vi "Update Fields Table for Spartan 3.0.vi"(8 "error in":errorcluster, 11 "Connection Refnum In":T1) -> (0 "error out":errorcluster, 3 "Connection Refnum Out":T1)   [LabVIEW 2011]
uses:
  Field Record.ctl
  Field DataTypes.ctl
  Field NextItem.ctl
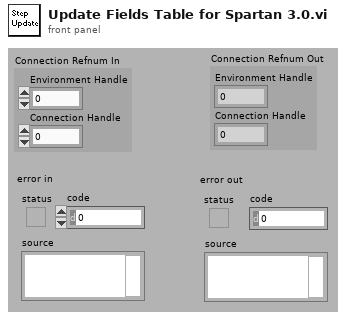
[diagram p1: front panel]
types:
  T1 = cluster{"Environment Handle":i32, "Connection Handle":i32}
  T2 = typedef "Field Record.ctl" = cluster{"ixField":i32, "iSequenceOrder":i32, "sxFieldId":string, "sxSequenceId":string, "sDisplayName":string, "sValue":string, "sUnits":string, "nDataType":T3, "nNextItem":T4, "fSystem":bool, "fSystemValue":bool, "fRequired":bool, "fSetAtTest":bool, "fTestField":bool, "fDeleted":bool, "fIndexed":bool, "fFreeList":bool}
  T3 = typedef "Field DataTypes.ctl" = enum32{"text", "numeric", "list", "timestamp", "boolean"}
  T4 = typedef "Field NextItem.ctl" = enum32{"Reset", "Retain", "Auto-Increment"}
  T5 = typedef "Connection Refnum.ctl" = cluster{"Environment Handle":i32, "Connection Handle":i32}
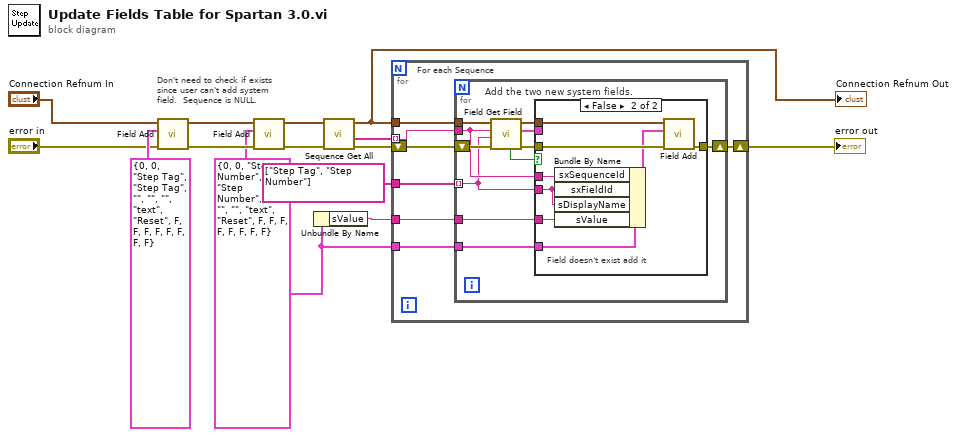
[diagram p0: block diagram]
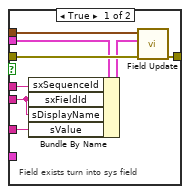
[diagram p2: hidden frame]
diagram:
  w6 = T2 {"ixField"=0, "iSequenceOrder"=0, "sxFieldId"="Step Number", "sxSequenceId"="Step Number", "sDisplayName"="", "sValue"="", "sUnits"="", "nDataType"=enum."text", "nNextItem"=enum."Reset", "fSystem"=FALSE, "fSystemValue"=FALSE, "fRequired"=FALSE, "fSetAtTest"=FALSE, "fTestField"=FALSE, "fDeleted"=FALSE, "fIndexed"=FALSE, "fFreeList"=FALSE} ("Field Record")
  # "Don't need to check if exists\nsince user can't add system\nfield.  Sequence is NULL."
  n1 = call "Field Add.vi"("error in (no error)"="error in", "Field Record"=T2 {"ixField"=0, "iSequenceOrder"=0, "sxFieldId"="Step Tag", "sxSequenceId"="Step Tag", "sDisplayName"="", "sValue"="", "sUnits"="", "nDataType"=enum."text", "nNextItem"=enum."Reset", "fSystem"=FALSE, "fSystemValue"=FALSE, "fRequired"=FALSE, "fSetAtTest"=FALSE, "fTestField"=FALSE, "fDeleted"=FALSE, "fIndexed"=FALSE, "fFreeList"=FALSE}, "Connection Refnum"="Connection Refnum In") -> ("error out"=w14:errorcluster, "Connection Refnum"=w13:T5)  [unwired: 1 in, 6 out]
  n2 = call "Field Add.vi"("error in (no error)"=w14, "Field Record"=w6, "Connection Refnum"=w13) -> ("error out"=w11:errorcluster, "Connection Refnum"=w12:T5)  [unwired: 1 in, 6 out]
  n3 = Unbundle By Name(w6) -> ("sValue"=w5:string)
  n4 = call "Sequence Get All.vi"("error in (no error)"=w11, "Connection Refnum"=w12) -> ("error out"=w9:errorcluster, "Sequence IDs"=w10:string[], "Connection Refnum"=w1:T5)  [unwired: 2 in, 5 out]
  "Connection Refnum Out" <- w1
  n5 = for {
    tunnel: w10 -> [w19] mode=indexing
    tunnel: w1 -> [w20]
    tunnel: string[] ["Step Tag", "Step Number"] -> [w18]
    shift-right: [w17] -> w2
    shift-left: w9 -> [w21]
    tunnel: w6 -> [w16]
    tunnel: w5 -> [w15]
    # "For each Sequence"
    n6 = for {
      tunnel: w20 -> [w31]
      tunnel: w19 -> [w27]
      tunnel: w18 -> [w25] mode=indexing
      shift-right: [w26] -> w17
      shift-left: w21 -> [w32]
      tunnel: w16 -> [w24]
      tunnel: w15 -> [w23]
      # "Add the two new system fields."
      n7 = call "Field Get Field.vi"("error in (no error)"=w32, "sFieldId or sDisplayName (\"\")"=w25, "sxSequenceId (\"\")"=w27, "Connection Refnum"=w31) -> ("error out"=w28:errorcluster, "Field"=w22:T2, "Connection Refnum"=w29:T5, "Data Present?"=w30:bool)  [unwired: 1 in, 3 out]
      n8 = case shown="False" w30 {
        tunnel: w29 -> [w40 w48]
        tunnel: w28 -> [w39 w47]
        tunnel: w27 -> [w37 w45]
        tunnel: [w36 w44] -> w26
        tunnel: w25 -> [w35 w43]
        tunnel: w24 -> [_ w42]
        tunnel: w23 -> [w34 w41]
        tunnel: w22 -> [w33 _]
        frame True {
          # "Field exists turn into sys field"
          n9 = Bundle By Name(cluster=w33, "sxSequenceId"=w37, "sxFieldId"=w35, "sDisplayName"=w35, "sValue"=w34) -> (w38:T2)
          n10 = call "Field Update.vi"("error in (no error)"=w39, "Field Record"=w38, "Connection Refnum"=w40) -> ("error out"=w36:errorcluster)  [unwired: 8 out]
        }
        frame False {
          # "Field doesn't exist add it"
          n11 = Bundle By Name(cluster=w42, "sxSequenceId"=w45, "sxFieldId"=w43, "sDisplayName"=w43, "sValue"=w41) -> (w46:T2)
          n12 = call "Field Add.vi"("error in (no error)"=w47, "Field Record"=w46, "Connection Refnum"=w48) -> ("error out"=w44:errorcluster)  [unwired: 1 in, 7 out]
        }
      }
    }
  }
  "error out" <- w2
